vi "Query Data as API String Arguments(variant).vi"(8 "error in":errorcluster, 9 "Setting Name":string, 11 "Internal Data":variant) -> (0 "error":errorcluster, 1 "Setting as String":string)   [LabVIEW 2017, in "API String Arguments Support.lvlib"]
uses:
  API String Arguments Support.lvlib
  <userlib>/_NEVSTOP/Communicable State Machine(CSM)/_Shared/CSM Shared.lvlib
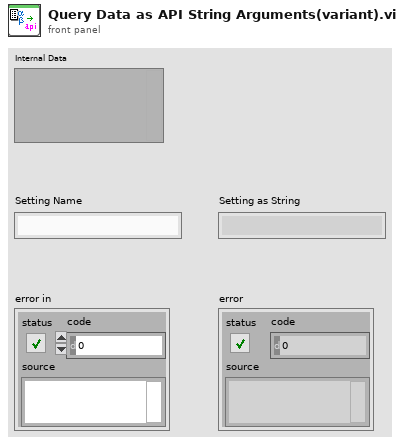
[diagram p1: front panel]
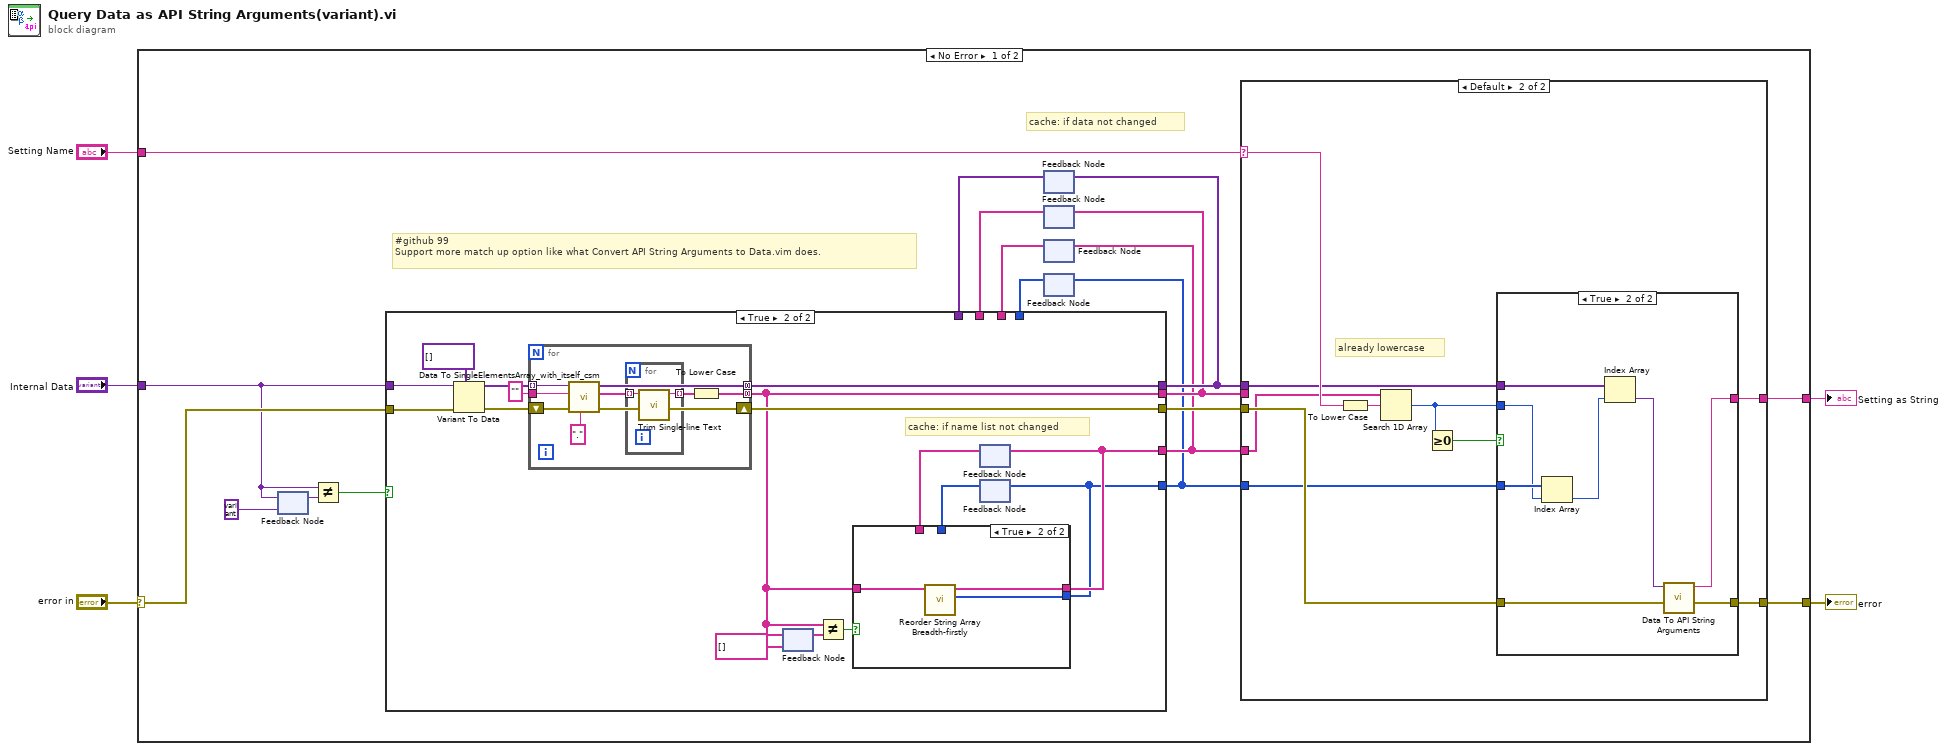
[diagram p0: block diagram]
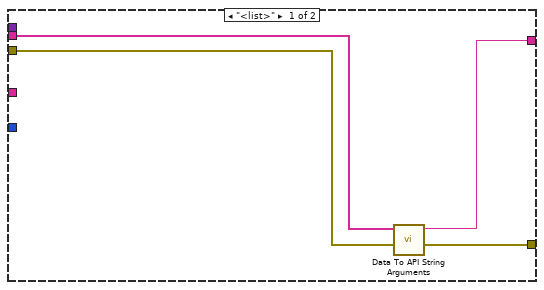
[diagram p4: hidden frame]
diagram:
  n1 = case shown="No Error" "error in" {
    selector: "error in" -> [w18 w83]
    tunnel: "Setting Name" -> [w22 _]
    tunnel: [w21 w83] -> w4
    tunnel: [w20 _] -> w3
    tunnel: "Internal Data" -> [w16 _]
    frame No Error {
      # "#github 99\nSupport more match up option like what Convert API String Arguments to Data.vim does."
      # "cache: if data not changed"
      n2 = feedback #1(variant ("Internal Data")) -> (w17:variant)
      n3 = feedback-in #1(w16) -> ()
      n4 = Not Equal?(x=w16, y=w17) -> (x != y?=w14:bool)
      n5 = feedback #2() -> (w12:variant[])  [unwired: 1 in]
      n6 = feedback #3() -> (w10:string[])  [unwired: 1 in]
      n7 = feedback #4() -> (w8:string[])  [unwired: 1 in]
      n8 = feedback #5() -> (w6:i32[])  [unwired: 1 in]
      n9 = case shown="True" w14 {
        tunnel: [w26 w42] -> w13
        tunnel: [w27 w41] -> w19
        tunnel: w18 -> [w27 w37]
        tunnel: [w24 w31] -> w9
        tunnel: [w23 w30] -> w7
        tunnel: [w25 w29] -> w11
        tunnel: w16 -> [_ w28]
        tunnel: w12 -> [w26 _]
        tunnel: w10 -> [w25 _]
        tunnel: w8 -> [w24 _]
        tunnel: w6 -> [w23 _]
        frame False {
        }
        frame True {
          # "cache: if name list not changed"
          n10 = Variant To Data(error in=w37, type=variant[] [] ("Array"), Variant=w28) -> (data=w39:variant[], error out=w38:errorcluster)
          n11 = for {
            tunnel: [w55] -> w42 mode=concatenating
            tunnel: [w49] -> w29 mode=concatenating
            tunnel: "" ("parentUrl") -> [w53]
            tunnel: w39 -> [w52] mode=indexing
            shift-right: [w54] -> w41
            shift-left: w38 -> [w57]
            n12 = call "Data To SingleElementsArray_with_itself_csm.vi"("Seperator(/)"=".", "error in (no error)"=w57, "parentUrl"=w53, "Cluster"=w52) -> ("error out"=w54:errorcluster, "Full NameList"=w50:string[], "DataElementArray"=w55:variant[])  [unwired: 5 in]
            n13 = for {
              tunnel: w50 -> [w59] mode=indexing
              tunnel: [w58] -> w51 mode=indexing
              n14 = call <userlib>:"Trim Single-line Text.vi"("single-line text"=w59) -> ("trimed text"=w58:string)  [unwired: 2 in]
            }
            n15 = To Lower Case(string=w51) -> (all lower case string=w49:string[])
          }
          n16 = feedback #6(string[] []) -> (w36:string[])
          n17 = feedback-in #6(w29) -> ()
          n18 = Not Equal?(x=w29, y=w36) -> (x != y?=w34:bool)
          n19 = feedback #7() -> (w32:string[])  [unwired: 1 in]
          n20 = feedback #8() -> (w33:i32[])  [unwired: 1 in]
          n21 = case shown="True" w34 {
            tunnel: w29 -> [_ w48]
            tunnel: [w44 w47] -> w31
            tunnel: [w45 w46] -> w30
            tunnel: w33 -> [w45 _]
            tunnel: w32 -> [w44 _]
            frame False {
            }
            frame True {
              n22 = call "Reorder String Array Breadth-firstly.vi"("Array 3"=w48) -> ("Indexs"=w46:i32[], "Array"=w47:string[])  [unwired: 9 in]
            }
          }
          n23 = feedback-in #7(w31) -> ()
          n24 = feedback-in #8(w30) -> ()
        }
      }
      n25 = feedback-in #2(w13) -> ()
      n26 = feedback-in #3(w11) -> ()
      n27 = feedback-in #4(w9) -> ()
      n28 = feedback-in #5(w7) -> ()
      n29 = case shown="Default" w22 {
        selector: w22 -> [_ w73]
        tunnel: [w61 w71] -> w21
        tunnel: [w63 w70] -> w20
        tunnel: w13 -> [_ w67]
        tunnel: w19 -> [w62 w66]
        tunnel: w9 -> [_ w65]
        tunnel: w7 -> [_ w64]
        tunnel: w11 -> [w60 _]
        frame "<list>" {
          n30 = call "Data To API String Arguments.vi"("error in (no error)"=w62, "data"=w60) -> ("error out"=w61:errorcluster, "String"=w63:string)  [unwired: 8 in]
        }
        frame Default {
          # "already lowercase"
          n31 = To Lower Case(string=w73) -> (all lower case string=w72:string)
          n32 = Search 1D Array(1D array=w65, element=w72) -> (index of element=w68:i32)  [unwired: 1 in]
          n33 = Greater Or Equal To 0?(x=w68) -> (x >= 0?=w69:bool)
          n34 = case shown="True" w69 {
            tunnel: w67 -> [_ w82]
            tunnel: w68 -> [_ w76]
            tunnel: w66 -> [w74 w80]
            tunnel: [w74 w78] -> w71
            tunnel: [_ w79] -> w70
            tunnel: w64 -> [_ w77]
            frame False {
            }
            frame True {
              n35 = Index Array(array=w77, index=w76) -> (element=w75:i32)
              n36 = Index Array(array=w82, index=w75) -> (element=w81:variant)
              n37 = call "Data To API String Arguments.vi"("error in (no error)"=w80, "data"=w81) -> ("error out"=w78:errorcluster, "String"=w79:string)  [unwired: 8 in]
            }
          }
        }
      }
    }
    frame Error {
    }
  }
  "Setting as String" <- w3
  "error" <- w4
